vi "Test Init.vi"(8 "error in (no error)":errorcluster, 11 "Address":string="09337296") -> (0 "error out":errorcluster, 3 "VISA resource name":refnum<visa-resource-name>)   [LabVIEW 2019, in "SR7270 Drivers.lvlib"]
uses:
  SR7270 Drivers.lvlib
  <vilib>/addons/_JKI Toolkits/Caraya/classes/Assert/Assert.lvclass
  <vilib>/addons/_JKI Toolkits/Caraya/classes/Test/Test.lvclass
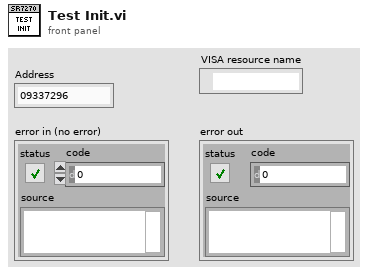
[diagram p1: front panel]
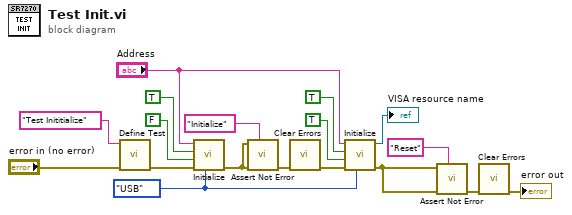
[diagram p0: block diagram]
diagram:
  w8 = enum16{"RS232", "USB", "Ethernet"}."USB" ("Interface")
  n1 = call <vilib>:"Define Test.vi"("error in (no error)"="error in (no error)", "Label (VI Title)"="Test Inititialize") -> ("error out"=w17:errorcluster)  [unwired: 9 in]
  n2 = call "Initialize.vi"("Interface"=w8, "error in (no error)"=w17, "reset"=FALSE, "ID query"=TRUE, "Address"="Address") -> ("error out"=w15:errorcluster)  [unwired: 5 in, 1 out]
  n3 = call <vilib>:"Assert Not Error.vi"("Label"="Initialize", "error in (no error)"=w15, "Not Error?"=w15) -> ("error out"=w13:errorcluster)  [unwired: 8 in]
  n4 = call <vilib>:"Clear Errors.vi"("error in (no error)"=w13) -> ("error out"=w5:errorcluster)  [unwired: 5 in, 1 out]
  n5 = call "Initialize.vi"("Interface"=w8, "error in (no error)"=w5, "reset"=TRUE, "ID query"=TRUE, "Address"="Address") -> ("error out"=w6:errorcluster, "VISA resource name out"=→"VISA resource name":refnum<visa-resource-name>)  [unwired: 5 in]
  n6 = call <vilib>:"Assert Not Error.vi"("Label"="Reset", "error in (no error)"=w6, "Not Error?"=w6) -> ("error out"=w7:errorcluster)  [unwired: 8 in]
  n7 = call <vilib>:"Clear Errors.vi"("error in (no error)"=w7) -> ("error out"=→"error out":errorcluster)  [unwired: 5 in, 1 out]
